vi "Remove_binaries.vi"() -> ()   [LabVIEW 2010]
panel:
  out "n_elem":i32
  in  "Separation Limit":dbl
  in  "Magnitude Difference Limit":dbl
  in  "USNO_data":string[][](array[string])
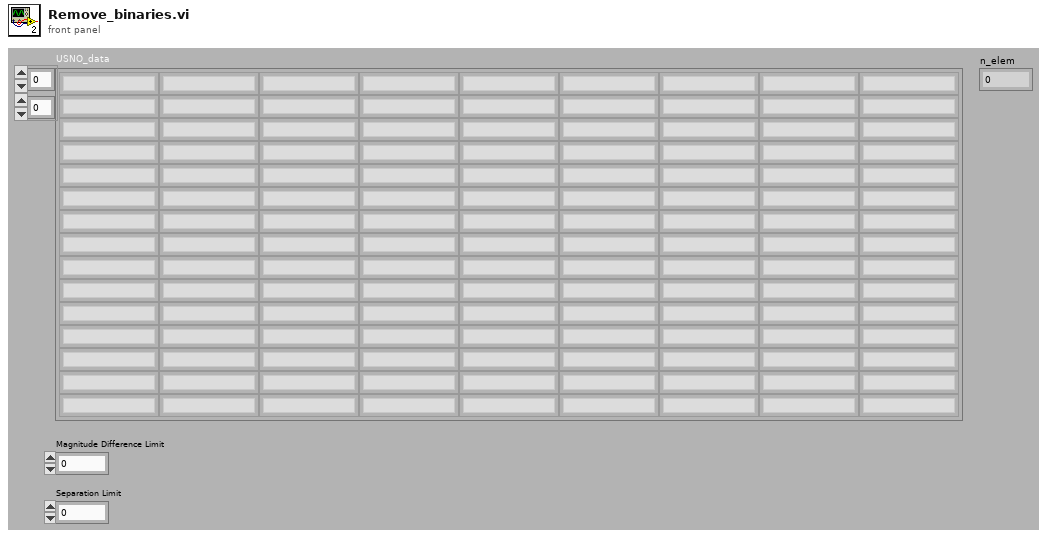
[diagram p1: front panel]
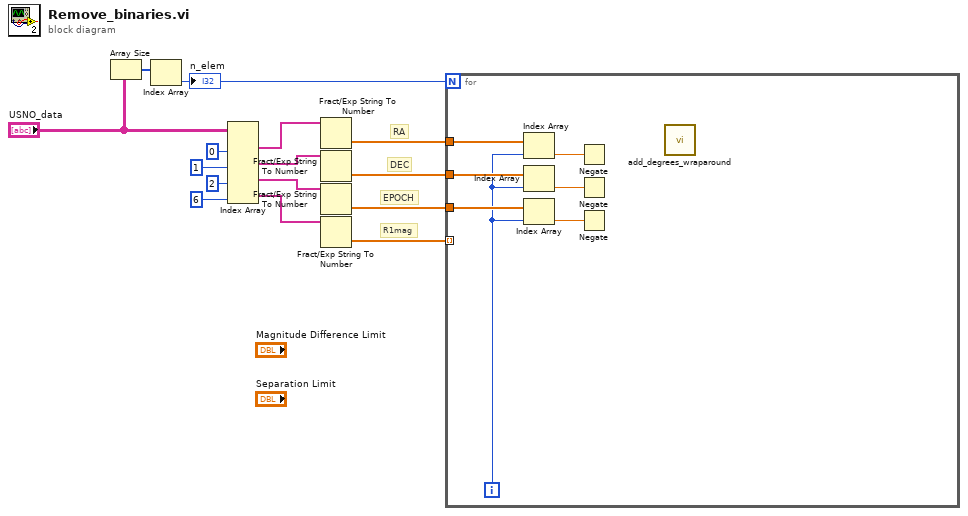
[diagram p0: block diagram]
diagram:
  # "R1mag"
  # "EPOCH"
  # "DEC"
  # "RA"
  n1 = Array Size(array="USNO_data") -> (size(s)=w14:i32[])
  n2 = Index Array(array=w14) -> (element=w9:i32)  [unwired: 1 in]
  "n_elem" <- w9
  n3 = Index Array(array="USNO_data", index (col) #1=0 ("disabled index (col)"), index (col) #2=1 ("index (col)"), index (col) #3=2 ("index (col)"), index (col) #4=6 ("index (col)")) -> (element #1=w8:string[], element #2=w7:string[], element #3=w6:string[], element #4=w5:string[])  [unwired: 4 in]
  n4 = Fract/Exp String To Number(string=w8) -> (number=w4:dbl[])  [unwired: 3 in, 1 out]
  n5 = Fract/Exp String To Number(string=w7) -> (number=w3:dbl[])  [unwired: 3 in, 1 out]
  n6 = Fract/Exp String To Number(string=w6) -> (number=w2:dbl[])  [unwired: 3 in, 1 out]
  n7 = Fract/Exp String To Number(string=w5) -> (number=w1:dbl[])  [unwired: 3 in, 1 out]
  n8 = for {
    N: w9 -> [_]
    tunnel: w4 -> [w16]
    tunnel: w3 -> [w22]
    tunnel: w2 -> [w21]
    tunnel: w1 -> [_] mode=indexing
    i -> [w20]
    n9 = Index Array(array=w16, index=w20) -> (element=w19:dbl)
    n10 = Index Array(array=w22, index=w20) -> (element=w18:dbl)
    n11 = Index Array(array=w21, index=w20) -> (element=w17:dbl)
    n12 = Negate(x=w19) -> ()  [unwired: 1 out]
    n13 = Negate(x=w18) -> ()  [unwired: 1 out]
    n14 = Negate(x=w17) -> ()  [unwired: 1 out]
    n15 = call "add_degrees_wraparound.vi"() -> ()  [unwired: 2 in, 1 out]
  }
